vi "Scripting_ConvertBaseClassToSubClass_UpdateCreate.vi"(8 "error in (no error)":errorcluster, 9 "NewViPath":path=path "C:/classes/NotBase_class/utils/NotBase_New.vi", 10 "Diagram":refnum<vi>, 11 "NewBaseCreate":refnum<vi>) -> (0 "error out":errorcluster)   [LabVIEW 2020]
doc: "Use this template to build a VI to use as a subVI."
uses:
  <vilib>/Utility/miscctls.llb/LVPointTypeDef.ctl
  <vilib>/Utility/miscctls.llb/LVPositionTypeDef.ctl
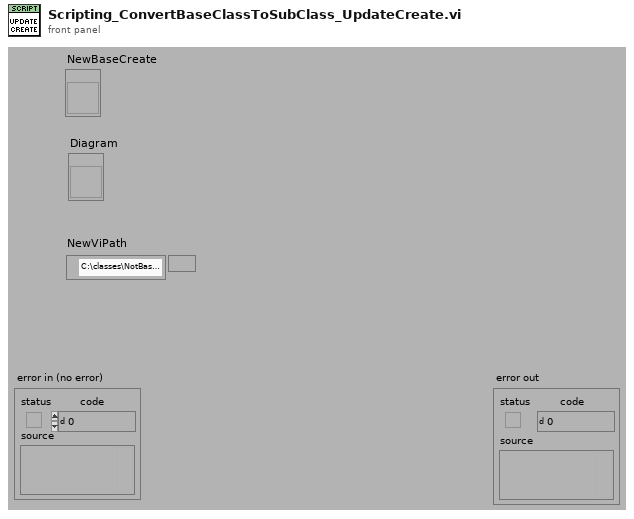
[diagram p1: front panel]
types:
  T1 = typedef "LVPositionTypeDef.ctl" = cluster{"Left":i32, "Top":i32}
  T2 = typedef "LVPointTypeDef.ctl" = cluster{"Horizontal":i16, "Vertical":i16}
  T3 = typedef "LVRectTypeDef.ctl" = cluster{"Left":i16, "Top":i16, "Right":i16, "Bottom":i16}
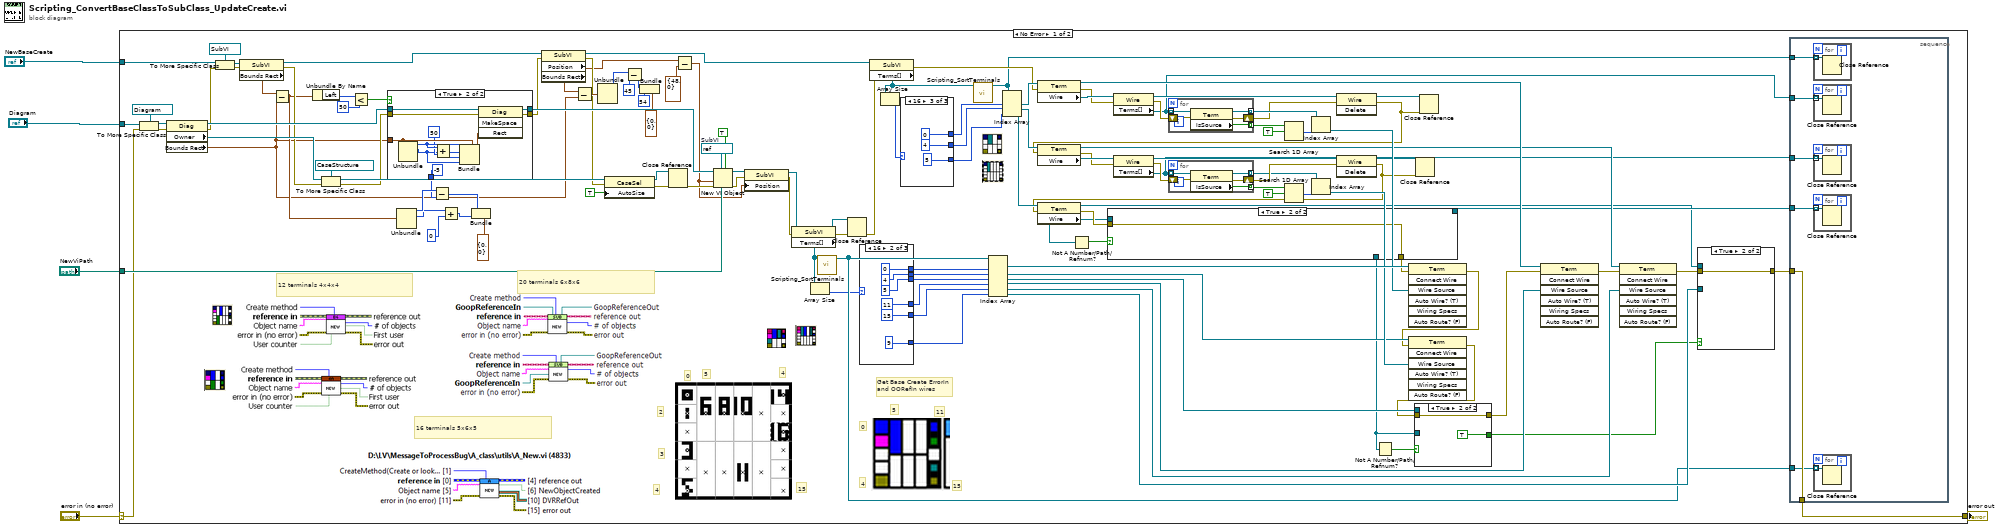
[diagram p0: block diagram]
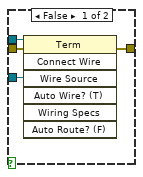
[diagram p2: hidden frame]
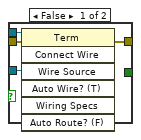
[diagram p3: hidden frame]
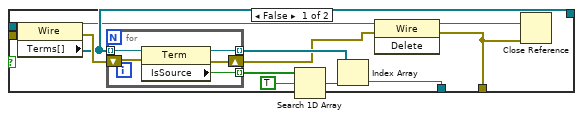
[diagram p4: hidden frame]
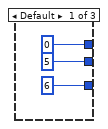
[diagram p5: hidden frame]
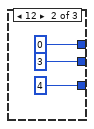
[diagram p6: hidden frame]
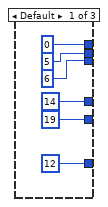
[diagram p7: hidden frame]
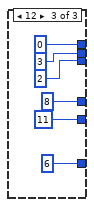
[diagram p8: hidden frame]
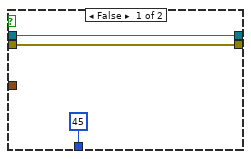
[diagram p9: hidden frame]
diagram:
  n1 = case shown="No Error" "error in (no error)" {
    selector: "error in (no error)" -> [w52 w225]
    tunnel: [w51 w225] -> w4
    tunnel: "NewBaseCreate" -> [w104 _]
    tunnel: "Diagram" -> [w124 _]
    tunnel: "NewViPath" -> [w116 _]
    frame No Error {
      w115 = refnum<vi> refnum  # SubVI
      # "15"
      # "11"
      # "5"
      # "4"
      # "0"
      # "3"
      # "2"
      # "4"
      # "15"
      # "4"
      # "0"
      # "5"
      # "16 terminals 5x6x5"
      # "20 terminals 6x8x6"
      # "12 terminals 4x4x4"
      # "Get Base Create ErrorIn\nand OORefIn wires"
      n2 = To More Specific Class(target class=refnum<vi> refnum ("Block Diagram"), reference=w124, error in=w52) -> (specific class reference=w132:refnum<vi>, error out=w123:errorcluster)
      n3 = property class="Diag"(reference=w132, error in=w123) -> (reference out=w122:refnum<vi>, error out=w103:errorcluster, "Owner"=w129:refnum<vi>, "Bounds Rect"=w39:T3)
      n4 = To More Specific Class(target class=refnum<vi> refnum ("Block Diagram"), reference=w104, error in=w103) -> (specific class reference=w101:refnum<vi>, error out=w102:errorcluster)
      n5 = property class="SubVI"(reference=w101, error in=w102) -> (reference out=w41:refnum<vi>, error out=w120:errorcluster, "Bounds Rect"=w118:T3)
      n6 = Subtract(x=w118, y=w39) -> (x-y=w111:T3)
      n7 = Unbundle By Name(w111) -> ("Left"=w121:i16)
      n8 = To More Specific Class(target class=refnum<vi> refnum ("Block Diagram"), reference=w129, error in=w120) -> (specific class reference=w131:refnum<vi>, error out=w119:errorcluster)
      n9 = Less?(x=w121, y=i16 50) -> (x < y?=w127:bool)
      n10 = case shown="True" w127 {
        tunnel: w122 -> [w212 w216]
        tunnel: w119 -> [w213 w217]
        tunnel: [w213 w224] -> w32
        tunnel: w39 -> [_ w221]
        tunnel: [w212 w215] -> w112
        tunnel: [i16 45 ("y") i16 -5 ("y")] -> w110
        frame False {
        }
        frame True {
          n11 = Unbundle(w221) -> ("Left"=w223:i16, "Top"=w219:i16)  [unwired: 2 out]
          n12 = Add(x=w223, y=i16 50) -> (x+y=w222:i16)
          n13 = Bundle(cluster=w221, "Left"=w223, "Top"=w219, "Right"=w222, "Bottom"=w219) -> (w218:T3)
          n14 = invoke class="Diag" method="MakeSpace"(reference=w216, error in=w217, "Rect"=w218) -> (reference out=w215:refnum<vi>, error out=w224:errorcluster)  [unwired: 1 in, 2 out]
        }
      }
      n15 = Unbundle(w111) -> ("Left"=w114:i16, "Top"=w108:i16)  [unwired: 2 out]
      n16 = Subtract(x=w114, y=w110) -> (x-y=w113:i16)
      n17 = Add(x=w108, y=i16 0) -> (x+y=w109:i16)
      n18 = Bundle(cluster=T2 {"Horizontal"=0, "Vertical"=0} ("relative position/next to refnum"), "Horizontal"=w113, "Vertical"=w109) -> ()  [unwired: 1 out]
      n19 = property class="SubVI"(reference=w41, error in=w32) -> (reference out=w40:refnum<vi>, error out=w33:errorcluster, "Position"=w12:T1, "Bounds Rect"=w13:T3)
      n20 = Subtract(x=w13, y=w39) -> (x-y=w38:T3)
      n21 = Unbundle(w38) -> ("Left"=w36:i16)  [unwired: 3 out]
      n22 = property class="CaseSel"(reference=w131, error in=w33, "AutoSize"=TRUE ("AutoSize To Fit Contents?")) -> (reference out=w60:refnum<vi>, error out=w62:errorcluster)
      n23 = Subtract(x=w36, y=i16 45) -> (x-y=w34:i16)
      n24 = Bundle(cluster=T2 {"Horizontal"=0, "Vertical"=0} ("relative position/next to refnum"), "Horizontal"=w34, "Vertical"=i16 54) -> ()  [unwired: 1 out]
      n25 = Close Reference(reference=w60, error in (no error)=w62) -> (error out=w61:errorcluster)
      n26 = Subtract(x=w12, y=T1 {"Left"=48, "Top"=0}) -> (x-y=w6:T1)
      n27 = New VI Object(vi object class=w115, auto wire? (F)=TRUE, owner refnum=w112, position/next to=w6, 6:w116, 8:w61) -> (object refnum=w10:refnum<vi>, 0:w9:errorcluster)  [unwired: 2 in]
      n28 = property class="SubVI"(reference=w10, error in=w9, "Position"=w6) -> (reference out=w8:refnum<vi>, error out=w7:errorcluster)
      n29 = property class="SubVI"(reference=w8, error in=w7) -> (reference out=w57:refnum<vi>, error out=w59:errorcluster, "Terms[]"=w30:refnum<vi>[])
      n30 = Array Size(array=w30) -> (size(s)=w29:i32)
      n31 = call "Scripting_SortTerminals.vi"("Terminals[]"=w30) -> ("TerminalsOut[]"=w31:refnum<vi>[])  [unwired: 8 in, 2 out]
      n32 = Close Reference(reference=w57, error in (no error)=w59) -> (error out=w58:errorcluster)
      n33 = case shown="16" w29 {
        tunnel: [14 ("index") 11 ("index") 8 ("index")] -> w73
        tunnel: [19 ("index") 15 ("index") 11 ("index")] -> w72
        tunnel: [12 ("index") 9 ("index") 6 ("index")] -> w47
        tunnel: [0 ("index") 0 ("index") 0 ("index")] -> w25
        tunnel: [6 ("index") 5 ("index") 2 ("index")] -> w28
        tunnel: [5 ("index") 4 ("index") 3 ("index")] -> w23
        frame Default {
        }
        frame 16 {
        }
        frame 12 {
        }
      }
      n34 = property class="SubVI"(reference=w40, error in=w58) -> (error out=w71:errorcluster, "Terms[]"=w21:refnum<vi>[])  [unwired: 1 out]
      n35 = Array Size(array=w21) -> (size(s)=w20:i32)
      n36 = case shown="16" w20 {
        tunnel: [0 ("index") 0 ("index") 0 ("index")] -> w24
        tunnel: [5 ("index") 3 ("index") 4 ("index")] -> w22
        tunnel: [6 ("index") 4 ("index") 5 ("index")] -> w26
        frame Default {
        }
        frame 12 {
        }
        frame 16 {
        }
      }
      n37 = call "Scripting_SortTerminals.vi"("Terminals[]"=w21) -> ("TerminalsOut[]"=w27:refnum<vi>[])  [unwired: 8 in, 2 out]
      n38 = Index Array(array=w31, index #1=w25, index #2=w23, index #3=w28, index #4=w73, index #5=w72, index #6=w47) -> (element #1=w89:refnum<vi>, element #2=w75:refnum<vi>, element #3=w74:refnum<vi>, element #4=w66:refnum<vi>, element #5=w63:refnum<vi>, element #6=w43:refnum<vi>)
      n39 = Index Array(array=w27, index #1=w24, index #2=w22, index #3=w26) -> (element #1=w100:refnum<vi>, element #2=w99:refnum<vi>, element #3=w98:refnum<vi>)
      n40 = property class="Term"(reference=w100, error in=w71) -> (reference out=w67:refnum<vi>, error out=w87:errorcluster, "Wire"=w97:refnum<vi>)
      n41 = property class="Wire"(reference=w97, error in=w87) -> (reference out=w91:refnum<vi>, error out=w92:errorcluster, "Terms[]"=w50:refnum<vi>[])
      n42 = for {
        tunnel: w50 -> [w210] mode=indexing
        tunnel: [w209] -> w96 mode=indexing
        tunnel: [w208] -> w93 mode=indexing
        shift-right: [w206] -> w90
        shift-left: w92 -> [w207]
        n43 = property class="Term"(reference=w210, error in=w207) -> (reference out=w208:refnum<vi>, error out=w206:errorcluster, "IsSource"=w209:bool)
      }
      n44 = Search 1D Array(1D array=w96, element=TRUE) -> (index of element=w94:i32)  [unwired: 1 in]
      n45 = Index Array(array=w93, index=w94) -> (element=w88:refnum<vi>)
      n46 = invoke class="Wire" method="Delete"(reference=w91, error in=w90) -> (reference out=w56:refnum<vi>, error out=w55:errorcluster)  [unwired: 1 in, 1 out]
      n47 = property class="Term"(reference=w99, error in=w55) -> (reference out=w64:refnum<vi>, error out=w78:errorcluster, "Wire"=w79:refnum<vi>)
      n48 = property class="Wire"(reference=w79, error in=w78) -> (reference out=w85:refnum<vi>, error out=w84:errorcluster, "Terms[]"=w49:refnum<vi>[])
      n49 = for {
        tunnel: w49 -> [w205] mode=indexing
        tunnel: [w204] -> w80 mode=indexing
        tunnel: [w203] -> w83 mode=indexing
        shift-right: [w201] -> w86
        shift-left: w84 -> [w202]
        n50 = property class="Term"(reference=w205, error in=w202) -> (reference out=w203:refnum<vi>, error out=w201:errorcluster, "IsSource"=w204:bool)
      }
      n51 = Search 1D Array(1D array=w80, element=TRUE) -> (index of element=w82:i32)  [unwired: 1 in]
      n52 = Index Array(array=w83, index=w82) -> (element=w76:refnum<vi>)
      n53 = invoke class="Wire" method="Delete"(reference=w85, error in=w86) -> (reference out=w54:refnum<vi>, error out=w53:errorcluster)  [unwired: 1 in, 1 out]
      n54 = property class="Term"(reference=w98, error in=w53) -> (reference out=w44:refnum<vi>, error out=w77:errorcluster, "Wire"=w19:refnum<vi>)
      n55 = Not A Number/Path/Refnum?(number/path/refnum=w19) -> (NaN/Path/Refnum?=w18:bool)
      n56 = case shown="True" w18 {
        tunnel: w77 -> [w151 w162]
        tunnel: [w150 _] -> w17
        tunnel: [w149 _] -> w48
        tunnel: [w145 w162] -> w42
        tunnel: w19 -> [w144 _]
        frame False {
          n57 = property class="Wire"(reference=w144, error in=w151) -> (reference out=w148:refnum<vi>, error out=w152:errorcluster, "Terms[]"=w149:refnum<vi>[])
          n58 = for {
            tunnel: w149 -> [w161] mode=indexing
            tunnel: [w160] -> w156 mode=indexing
            tunnel: [w159] -> w153 mode=indexing
            shift-right: [w157] -> w146
            shift-left: w152 -> [w158]
            n59 = property class="Term"(reference=w161, error in=w158) -> (reference out=w159:refnum<vi>, error out=w157:errorcluster, "IsSource"=w160:bool)
          }
          n60 = Search 1D Array(1D array=w156, element=TRUE) -> (index of element=w154:i32)  [unwired: 1 in]
          n61 = Index Array(array=w153, index=w154) -> (element=w150:refnum<vi>)
          n62 = invoke class="Wire" method="Delete"(reference=w148, error in=w146) -> (reference out=w147:refnum<vi>, error out=w145:errorcluster)  [unwired: 1 in, 1 out]
          n63 = Close Reference(reference=w147, error in (no error)=w145) -> ()  [unwired: 1 out]
        }
        frame True {
        }
      }
      n64 = Not A Number/Path/Refnum?(number/path/refnum=w17) -> (NaN/Path/Refnum?=w16:bool)
      n65 = invoke class="Term" method="Connect Wire"(reference=w89, error in=w42, "Wire Source"=w88) -> (error out=w70:errorcluster)  [unwired: 4 in, 6 out]
      n66 = invoke class="Term" method="Connect Wire"(reference=w75, error in=w70, "Wire Source"=w76) -> (error out=w69:errorcluster)  [unwired: 4 in, 6 out]
      n67 = case shown="True" w16 {
        tunnel: w74 -> [w141 _]
        tunnel: w69 -> [w140 w143]
        tunnel: [w139 w143] -> w68
        tunnel: w17 -> [w138 _]
        tunnel: [_ TRUE] -> w15
        frame False {
          n68 = invoke class="Term" method="Connect Wire"(reference=w141, error in=w140, "Wire Source"=w138) -> (error out=w139:errorcluster)  [unwired: 4 in, 6 out]
        }
        frame True {
        }
      }
      n69 = Close Reference(reference=w54, error in (no error)=w53) -> ()  [unwired: 1 out]
      n70 = Close Reference(reference=w56, error in (no error)=w55) -> ()  [unwired: 1 out]
      n71 = invoke class="Term" method="Connect Wire"(reference=w67, error in=w68, "Wire Source"=w66) -> (error out=w65:errorcluster)  [unwired: 4 in, 6 out]
      n72 = invoke class="Term" method="Connect Wire"(reference=w64, error in=w65, "Wire Source"=w63) -> (error out=w46:errorcluster)  [unwired: 4 in, 6 out]
      n73 = case shown="True" w15 {
        tunnel: w46 -> [w136 w137]
        tunnel: [w135 w137] -> w45
        tunnel: w44 -> [w134 _]
        tunnel: w43 -> [w133 _]
        frame False {
          n74 = invoke class="Term" method="Connect Wire"(reference=w134, error in=w136, "Wire Source"=w133) -> (error out=w135:errorcluster)  [unwired: 4 in, 6 out]
        }
        frame True {
        }
      }
      n75 = stacked-sequence {
        tunnel: [w195] -> w51
        tunnel: w45 -> [w195]
        tunnel: w27 -> [w194]
        tunnel: w31 -> [w193]
        tunnel: w50 -> [w192]
        tunnel: w49 -> [w191]
        tunnel: w48 -> [w190]
        frame #0 {
          n76 = for {
            tunnel: w194 -> [w200] mode=indexing
            n77 = Close Reference(reference=w200) -> ()  [unwired: 1 in, 1 out]
          }
          n78 = for {
            tunnel: w192 -> [w198] mode=indexing
            n79 = Close Reference(reference=w198) -> ()  [unwired: 1 in, 1 out]
          }
          n80 = for {
            tunnel: w191 -> [w197] mode=indexing
            n81 = Close Reference(reference=w197) -> ()  [unwired: 1 in, 1 out]
          }
          n82 = for {
            tunnel: w190 -> [w196] mode=indexing
            n83 = Close Reference(reference=w196) -> ()  [unwired: 1 in, 1 out]
          }
          n84 = for {
            tunnel: w193 -> [w199] mode=indexing
            n85 = Close Reference(reference=w199) -> ()  [unwired: 1 in, 1 out]
          }
        }
      }
    }
    frame Error {
    }
  }
  "error out" <- w4
